vi "2P_AdapUprite_Linlin.vi"() -> ()   [LabVIEW 2015] (continued)
                                n2049 = call "waveformparamsv2.vi"("command"="add DO", "add DO"=w5235) -> ()  [unwired: 3 in, 3 out]
                                }
                                frame #2 {
                                n2050 = call "waveformsDObuffer.vi"("command"="get") -> ("DO wf out"=w5240:digitalwaveform[])  [unwired: 1 in]
                                n2051 = Build Array (concatenate)(w5240, w5237) -> (w5239:digitalwaveform[])
                                n2052 = call "waveformsDObuffer.vi"("DO wf in"=w5239, "command"="set") -> ()  [unwired: 1 out]
                                }
                                }
                                }
                                frame 0 {
                                n2053 = stacked-sequence {
                                seq-local: [w5248 _ _] -> [_ w5256 w5273]
                                tunnel: w5245 -> [_ _ _]
                                tunnel: w5244 -> [_ _ _]
                                tunnel: w5243 -> [_ w5253 _]
                                tunnel: w5242 -> [_ _ w5272]
                                frame #0 {
                                n2054 = call "configuration_2P_Linlin.vi"("command"="get") -> ("config out"=w5246:T14)  [unwired: 2 in, 1 out]
                                n2055 = Unbundle By Name(w5246) -> ("LT timestamp"=w5249:u32)
                                n2056 = call "2pparameters.vi"("command"="get") -> ("params out"=w5252:T12)  [unwired: 1 in]
                                n2057 = Unbundle By Name(w5252) -> ("aDO"=w5250:u32[])
                                n2058 = Search 1D Array(1D array=w5250, element=w5249) -> (index of element=w5248:i32)  [unwired: 1 in]
                                }
                                frame #1 {
                                n2059 = local read "Measurement"() -> (w5255:T4)
                                n2060 = To Unsigned Long Integer(number=w5255) -> (unsigned 32bit integer=w5254:u32)
                                n2061 = case shown="5..7" w5254 {
                                tunnel: w5256 -> [_ w5260]
                                tunnel: w5253 -> [_ w5257]
                                frame 0..4, Default {
                                }
                                frame 5..7 {
                                n2062 = Index Array(array=w5257, index=0) -> (element=w5258:T21)
                                n2063 = call "waveformparamsv2.vi"("command"="get") -> ("Params out"=w5263:T17)  [unwired: 4 in, 2 out]
                                n2064 = in-place {
                                in-place-border: w5260 -> [w5267]
                                in-place-border: w5258 -> [w5265]
                                n2065 = in-place-cluster #43(w5263) -> ("DO parameters"=w5268:T20)
                                n2066 = in-place {
                                in-place-border: w5265 -> [w5269]
                                n2067 = in-place-array #44(w5268, w5267) -> ()  [unwired: 1 out]
                                n2068 = in-place-array #44(w5269) -> (w5266:T20)  [unwired: 1 out]
                                }
                                n2069 = in-place-cluster #43("DO parameters"=w5266) -> (w5261:T17)
                                }
                                n2070 = call "waveformparamsv2.vi"("command"="set", "Params in"=w5261) -> ()  [unwired: 3 in, 3 out]
                                }
                                }
                                }
                                frame #2 {
                                n2071 = local read "Measurement"() -> (w5271:T4)
                                n2072 = To Unsigned Long Integer(number=w5271) -> (unsigned 32bit integer=w5270:u32)
                                n2073 = case shown="5..7" w5270 {
                                tunnel: w5273 -> [_ w5277]
                                tunnel: w5272 -> [_ w5275]
                                frame 0..4, Default {
                                }
                                frame 5..7 {
                                n2074 = Index Array(array=w5275, index=0) -> (element=w5274:digitalwaveform)
                                n2075 = call "waveformsDObuffer.vi"("command"="get") -> ("DO wf out"=w5279:digitalwaveform[])  [unwired: 1 in]
                                n2076 = Replace Array Subset(array=w5279, new element=w5274, index=w5277) -> (w5281:digitalwaveform[])
                                n2077 = call "waveformsDObuffer.vi"("DO wf in"=w5281, "command"="set") -> ()  [unwired: 1 out]
                                }
                                }
                                }
                                }
                                }
                                }
                              }
                              frame #4 {
                                n2078 = call "Used AO lines.vi"() -> ("used AO names"=w5284:string[], "used AO lines"=w5282:tag[])  [unwired: 2 in]
                                n2079 = control-ref of="Analog Lines Plot"() -> (w5283:refnum<vi>)
                                n2080 = control-ref of="Digital Lines Plot"() -> (w5285:refnum<vi>)
                                n2081 = call "Used DO lines.vi"() -> ("used DO names"=w5286:string[], "used DO lines"=w5287:tag[])  [unwired: 2 in]
                                n2082 = local write "Analog Used Lines"(w5282) -> ()
                                n2083 = local write "Analog Used Names"(w5284) -> ()
                                n2084 = local write "Digital Used Lines"(w5287) -> ()
                                n2085 = local write "Digital Used Names"(w5286) -> ()
                                n2086 = call "prepDOWaveplot.vi"("DigitalGraph in"=w5285, "used DO names"=w5286) -> ()  [unwired: 1 in]
                                n2087 = call "prepAOWaveplot.vi"("WaveformGraph in"=w5283, "Analog Used Names"=w5284) -> ()  [unwired: 1 in]
                              }
                              frame #5 {
                                # "source of crashing?"
                                n2088 = local read "Meastab"() -> (w5302:enum32{"X-Y Image", "Linescan", "Timetrace"})
                                n2089 = property on="refwf" class="Ring (strict)"() -> ("RingText.Text"=w5299:string)  [unwired: 2 in, 2 out]
                                n2090 = case shown="\"Timetrace\"" w5302 {
                                tunnel: [w5304 w5305] -> w5303
                                frame "X-Y Image", Default {
                                n2091 = local read "Sampling rate"() -> (w5304:dbl)
                                }
                                frame "Timetrace" {
                                n2092 = local read "srateAODOtt"() -> (w5305:dbl)
                                }
                                }
                                n2093 = call "waveformsAObuffer.vi"("command"="get") -> ("AO wf out"=w5290:waveform(dbl)[])  [unwired: 1 in]
                                n2094 = local read "wavdet"() -> (w5300:bool)
                                n2095 = call "waveformsDObuffer.vi"("command"="get") -> ("DO wf out"=w5294:digitalwaveform[])  [unwired: 1 in]
                                n2096 = call "correctwaveformsizetemp.vi"("new sampling frequency (Hz)"=w5303, "start"=FALSE, "reference waveforms to"=w5299, "Analog waveforms in"=w5290, "stop"=TRUE, "Digital waveforms in"=w5294) -> ("analog wf out"=w5296:waveform(dbl)[], "Digital wf out"=w5298:digitalwaveform[], "measpoints"=w5301:i32)
                                n2097 = local write "Analog Lines Plot"(w5296) -> ()
                                n2098 = call "GetNumCamFramesv2.vi"("Digital Waveform Graph"=w5298) -> ("Numeric"=w5297:i32)  [unwired: 10 in]
                                n2099 = local write "Digital Lines Plot"(w5298) -> ()
                                n2100 = call "waveformsDObuffer.vi"("DO wf in"=w5298, "command"="set") -> ()  [unwired: 1 out]
                                n2101 = call "waveformsAObuffer.vi"("AO wf in"=w5296, "command"="set") -> ()  [unwired: 1 out]
                                n2102 = local write "Total Camera Frames"(w5297) -> ()
                                n2103 = case shown="True" w5300 {
                                tunnel: w5301 -> [_ w5306]
                                frame False {
                                }
                                frame True {
                                n2104 = local write "# of frames"(w5306) -> ()
                                }
                                }
                              }
                            }
                          }
                          frame #9 {
                            w5316 = FALSE ("Value (Signaling)")
                            # "Save parameters, reset system..."
                            n2105 = local read "save\ndata"() -> (w5311:bool)
                            n2106 = case shown="True" w5311 {
                              tunnel: w5310 -> [_ w5323]
                              frame False {
                              }
                              frame True {
                                n2107 = call "closebinaryfiles.vi"() -> ()  [unwired: 12 in]
                                n2108 = local read "filename prefix"() -> (w5324:string)
                                n2109 = local read "data dir"() -> (w5325:path)
                                n2110 = disable-structure shown="Disabled" {
                                disable-tunnel: w5324 -> [w5328 _]
                                disable-tunnel: w5325 -> [w5327 _]
                                disable-tunnel: w5323 -> [w5326 _]
                                frame Disabled {
                                n2111 = call "saveparams.vi"("timestamp"=w5326, "filename prefix in"=w5328, "data dir in"=w5327) -> ()  [unwired: 1 in]
                                }
                                frame Enabled {
                                }
                                }
                                n2112 = call "saveparams_andscanpattern.vi"("timestamp"=w5323, "filename prefix in"=w5324, "data dir in"=w5325) -> ()  [unwired: 1 in]
                              }
                            }
                            n2113 = call "2pparameters.vi"("command"="get") -> ("params out"=w5307:T12)  [unwired: 1 in]
                            n2114 = Unbundle By Name(w5307) -> ("auto OD"=w5308:bool)
                            n2115 = case shown="True" w5308 {
                              frame False {
                              }
                              frame True {
                                n2116 = call "configuration_2P_Linlin.vi"("command"="get") -> ("config out"=w5317:T14)  [unwired: 2 in, 1 out]
                                n2117 = call "2pparameters.vi"("command"="get") -> ("params out"=w5322:T12)  [unwired: 1 in]
                                n2118 = Unbundle By Name(w5317) -> ("contour OD"=w5319:u16)
                                n2119 = Unbundle By Name(w5322) -> ("ODfilt"=w5320:u16)
                                n2120 = call "filterwheelcontrol_nothorlabslib.vi"("Current OD filt"=w5319, "New ODfilt"=w5320) -> ()  [unwired: 1 in]
                              }
                            }
                            n2121 = property on="Start" class="Bool (strict)"("Val(Sgnl)"=w5316) -> ()  [unwired: 2 in, 2 out]
                            n2122 = property on="Start" class="Bool (strict)"("Visible"=TRUE, "DisabledEnum"=T7."Enabled" ("Disabled")) -> ()  [unwired: 2 in, 2 out]
                            n2123 = property on="Stop" class="Bool (strict)"("Val(Sgnl)"=w5316) -> ()  [unwired: 2 in, 2 out]
                            n2124 = property on="Stop" class="Bool (strict)"("Visible"=FALSE, "DisabledEnum"=T7."Disabled" ("Disabled")) -> ()  [unwired: 2 in, 2 out]
                          }
                          frame #10 {
                            w5331 = T24 2 items=["no dialog", "OK message", "continue or stop message", "OK message + warnings", "continue/stop + warnings"] ("type of dialog (OK msg:1)")
                            # "Error Handling"
                            n2125 = call "displayerrors.vi"() -> ("error IO"=w5332:errorcluster)
                            n2126 = call <vilib>:"General Error Handler.vi"("type of dialog (OK msg:1)"=w5331, "error in (no error)"=w5332) -> ("error out"=w5330:errorcluster)  [unwired: 9 in, 4 out]
                            n2127 = call <vilib>:"Clear Errors.vi"("error in (no error)"=w5330) -> ("error out"=w5329:errorcluster)  [unwired: 5 in, 1 out]
                            n2128 = call "seterrors.vi"("error IO"=w5329) -> ()
                          }
                        }
                      }
                    }
                  }
                  frame "Lifetime (point)" {
                    # "Not really used"
                    # "Disabled for conversion to 64 bit"
                    n2129 = disable-structure shown="Disabled" {
                      frame Disabled {
                        n2130 = stacked-sequence {
                          frame #0 {
                            w5353 = 0.1 ("Y Scale.Range:Minimum")
                            w5354 = 0.0 ("X Scale.Range:Minimum")
                            # "get from syncrate"
                            n2131 = local read item#-1() -> (w5338)
                            n2132 = local read "Vx-ref"() -> (w5350:dbl)
                            n2133 = local read "Vy-ref"() -> (w5351:dbl)
                            n2134 = call "2pparameters.vi"("command"="get") -> ("params out"=w5336:T12)  [unwired: 1 in]
                            n2135 = Scale By Power Of 2(n=w5338, x=1.0 ("Y Scale.Range:Minimum")) -> (x*2^n=w5347:dbl)
                            n2136 = call "setposition.vi"("Vy"=w5351, "Vx"=w5350) -> ()  [unwired: 1 in]
                            n2137 = Unbundle By Name(w5336) -> ("autoshutter"=w5337:bool, "aAS"=w5334:u32[])
                            n2138 = Multiply(x=3000.0 ("Y Scale.Range:Minimum"), y=w5347) -> (x*y=w5345:dbl)
                            n2139 = Compound Arithmetic op=MULTIPLY(12.5 ("x"), invert 3200.0 ("X Scale.Offset and Multiplier:Multiplier"), w5347) -> (w5346:dbl)
                            n2140 = case shown="True" w5337 {
                              tunnel: w5334 -> [_ w5363]
                              frame False {
                              }
                              frame True {
                                n2141 = call "shuttercontrol_multi.vi"("Autoshutter Chans"=w5363, "command"="open") -> ()  [unwired: 1 in, 1 out]
                              }
                            }
                            n2142 = call "lifetimeparameters.vi"("command"="get") -> ("Params out"=w5342:T22)  [unwired: 1 in]
                            n2143 = Bundle By Name(cluster=w5342, "Bin size"=w5338) -> (w5343:T22)
                            n2144 = call "lifetimeparameters.vi"("Params in"=w5343, "command"="set") -> ()  [unwired: 1 out]
                            n2145 = call "2pparameters.vi"("command"="get") -> ("params out"=w5358:T12)  [unwired: 1 in]
                            n2146 = Bundle By Name(cluster=w5358, "type"="Lifetime (point)") -> (w5356:T12)
                            n2147 = property on="Stop" class="Bool (strict)"("Visible"=TRUE, "DisabledEnum"=T7."Enabled" ("Disabled")) -> ()  [unwired: 2 in, 2 out]
                            n2148 = property on="Start" class="Bool (strict)"("Visible"=FALSE, "DisabledEnum"=T7."Disabled and Grayed Out" ("Disabled")) -> ()  [unwired: 2 in, 2 out]
                            n2149 = call "2pparameters.vi"("Params in"=w5356, "command"="set") -> ()  [unwired: 1 out]
                          }
                          frame #1 {
                            n2150 = call "setup.vi"() -> ()  [unwired: 1 in]
                          }
                          frame #2 {
                            # "main loop"
                            n2151 = call "lifetimeparameters.vi"("command"="get") -> ("Params out"=w5369:T22)  [unwired: 1 in]
                            n2152 = Unbundle By Name(w5369) -> ("devidx"=w5367:i32)
                            n2153 = for {
                              N: 10000 -> [_]
                              tunnel: [w5370] -> w5365 mode=indexing
                              i -> [w5370]
                            }
                            n2154 = while {
                              tunnel: w5367 -> [w5374]
                              tunnel: w5365 -> [w5371]
                              i -> [w5372]
                              stop <- w5376 stop-if-true
                              n2155 = Increment(x=w5372) -> (x+1=w5373:i32)
                              n2156 = dll-call lib="phlib.dll" fn="_PH_GetCountRate@8" label="PH_GetCountRate"("devidx"=w5374, "channel"=0) -> (w5375:i32)  [unwired: 5 in, 2 out]
                              n2157 = stacked-sequence {
                                seq-local: [_ _ w5382 _ _] -> [_ _ _ w5395 _]
                                seq-local: [_ _ w5381 _ _] -> [_ _ _ w5394 _]
                                seq-local: [_ w5380 _ _ _] -> [_ _ w5383 _ _]
                                tunnel: w5375 -> [_ _ _ w5402 _]
                                tunnel: w5371 -> [_ _ _ w5392 _]
                                frame #0 {
                                n2158 = call "start_binned.vi"() -> ()  [unwired: 1 in]
                                }
                                frame #1 {
                                n2159 = call "get-histogram.vi"() -> ("Histogram"=w5380:u32[])  [unwired: 1 out]
                                }
                                frame #2 {
                                n2160 = Search 1D Array(1D array=w5383, element=u32 0) -> (index of element=w5381:i32)  [unwired: 1 in]
                                n2161 = Multiply(x=w5381, y=0.99) -> (x*y=w5387:dbl)
                                n2162 = Array Subset(array=w5383, index=0, length=w5387) -> (w5390:u32[])
                                n2163 = Array Max & Min(array=w5390) -> (max index (indices)=w5384:i32)  [unwired: 3 out]
                                n2164 = Split 1D Array(array=w5390, index=w5384) -> (second subarray=w5386:u32[])  [unwired: 1 out]
                                n2165 = Array Max & Min(array=w5386) -> (min index (indices)=w5385:i32)  [unwired: 3 out]
                                n2166 = Split 1D Array(array=w5386, index=w5385) -> (first subarray=w5382:u32[])  [unwired: 1 out]
                                }
                                frame #3 {
                                n2167 = Array Size(array=w5395) -> (size(s)=w5397:i32)
                                n2168 = Array Subset(array=w5392, index=0, length=w5397) -> (w5396:i32[])
                                n2169 = Compound Arithmetic op=MULTIPLY(1000000000.0 ("value"), invert w5402, invert w5394, w5396) -> (w5393:dbl[])
                                n2170 = call <vilib>:"Exponential Fit.vi"("Y"=w5395, "X"=w5393) -> ("damping"=w5399:dbl)  [unwired: 8 in, 5 out]
                                n2171 = Divide(x=-1.0 ("y"), y=w5399) -> (x/y=w5403:dbl)
                                }
                                frame #4 {
                                n2172 = local read "downright"() -> (w5409:bool)
                                n2173 = local read "downleft"() -> (w5411:bool)
                                n2174 = local read "upright"() -> (w5407:bool)
                                n2175 = local read "upleft"() -> (w5405:bool)
                                n2176 = local read "down"() -> (w5410:bool)
                                n2177 = local read "right"() -> (w5408:bool)
                                n2178 = local read "left"() -> (w5412:bool)
                                n2179 = local read "up"() -> (w5406:bool)
                                n2180 = Compound Arithmetic op=OR(w5405, w5406, w5407, w5408, w5409, w5410, w5411, w5412) -> (w5404:bool)
                                n2181 = case shown="True" w5404 {
                                frame False {
                                }
                                frame True {
                                n2182 = stacked-sequence {
                                frame #0 {
                                n2183 = local read "downright"() -> (w5414:bool)
                                n2184 = local read "downleft"() -> (w5416:bool)
                                n2185 = local read "BigSmall"() -> (w5413:bool)
                                n2186 = local read "upright"() -> (w5418:bool)
                                n2187 = local read "upleft"() -> (w5421:bool)
                                n2188 = local read "down"() -> (w5417:bool)
                                n2189 = local read "right"() -> (w5419:bool)
                                n2190 = local read "left"() -> (w5415:bool)
                                n2191 = local read "up"() -> (w5420:bool)
                                n2192 = call "movestageparams.vi"("command"="get") -> ("Params out"=w5424:T23)  [unwired: 1 in]
                                n2193 = Bundle By Name(cluster=w5424, "upleft"=w5421, "up"=w5420, "upright"=w5418, "right"=w5419, "downright"=w5414, "down"=w5417, "downleft"=w5416, "left"=w5415, "Bigsmall"=w5413) -> (w5425:T23)
                                n2194 = call "movestageparams.vi"("Params in"=w5425, "command"="set") -> ()  [unwired: 1 out]
                                }
                                frame #1 {
                                n2195 = call "movestage.vi"() -> ()  [unwired: 12 in]
                                }
                                frame #2 {
                                w5426 = FALSE ("OK Button")
                                w5427 = FALSE ("OK Button")
                                n2196 = property on="down" class="Bool (strict)"("Value"=w5427) -> ()  [unwired: 2 in, 2 out]
                                n2197 = property on="up" class="Bool (strict)"("Value"=w5427) -> ()  [unwired: 2 in, 2 out]
                                n2198 = property on="right" class="Bool (strict)"("Value"=w5427) -> ()  [unwired: 2 in, 2 out]
                                n2199 = property on="left" class="Bool (strict)"("Value"=w5427) -> ()  [unwired: 2 in, 2 out]
                                n2200 = property on="upleft" class="Bool (strict)"("Value"=w5426) -> ()  [unwired: 2 in, 2 out]
                                n2201 = property on="upright" class="Bool (strict)"("Value"=w5426) -> ()  [unwired: 2 in, 2 out]
                                n2202 = property on="downleft" class="Bool (strict)"("Value"=w5426) -> ()  [unwired: 2 in, 2 out]
                                n2203 = property on="downright" class="Bool (strict)"("Value"=w5426) -> ()  [unwired: 2 in, 2 out]
                                }
                                }
                                }
                                }
                                }
                              }
                              n2204 = dll-call lib="phlib.dll" fn="_PH_GetCountRate@8" label="PH_GetCountRate"("devidx"=w5374, "channel"=1) -> (w5379:i32)  [unwired: 5 in, 2 out]
                              n2205 = local read "Stop"() -> (w5376:bool)
                              n2206 = local write "points recorded"(w5373) -> ()
                            }
                          }
                          frame #3 {
                            w5436 = FALSE ("Value (Signaling)")
                            n2207 = call "2pparameters.vi"("command"="get") -> ("params out"=w5430:T12)  [unwired: 1 in]
                            n2208 = Unbundle By Name(w5430) -> ("autoshutter"=w5431:bool, "aAS"=w5428:u32[])
                            n2209 = case shown="True" w5431 {
                              tunnel: w5428 -> [_ w5437]
                              frame False {
                              }
                              frame True {
                                n2210 = call "shuttercontrol_multi.vi"("Autoshutter Chans"=w5437, "command"="close") -> ()  [unwired: 1 in, 1 out]
                              }
                            }
                            n2211 = property on="Start" class="Bool (strict)"("Val(Sgnl)"=w5436) -> ()  [unwired: 2 in, 2 out]
                            n2212 = property on="Start" class="Bool (strict)"("Visible"=TRUE, "DisabledEnum"=T7."Enabled" ("Disabled")) -> ()  [unwired: 2 in, 2 out]
                            n2213 = property on="Stop" class="Bool (strict)"("Val(Sgnl)"=w5436) -> ()  [unwired: 2 in, 2 out]
                            n2214 = property on="Stop" class="Bool (strict)"("Visible"=FALSE, "DisabledEnum"=T7."Disabled" ("Disabled")) -> ()  [unwired: 2 in, 2 out]
                          }
                        }
                      }
                      frame Enabled {
                      }
                    }
                    n2215 = local write "64bit disabled"(TRUE ("64bit disabled")) -> ()
                  }
                }
              }
            }
          }
          event "avpp", "Angle ref", "xpixels ref", "Vx-min ref", "Vx-max ref", "ypixels ref", "Vy-min ref", "Vy-max ref", "ROI Type", "Sampling rate": Value Change {
            n2216 = event-data() -> ()  [unwired: 1 in, 6 out]
            n2217 = local read "avpp"() -> (w5456:i32)
            n2218 = local read "Angle ref"() -> (w5455:dbl)
            n2219 = local read "ROI Type"() -> (w5454:u16)
            n2220 = local read "xpixels ref"() -> (w5451:i32)
            n2221 = local read "Vx-min ref"() -> (w5450:dbl)
            n2222 = local read "Vx-max ref"() -> (w5449:dbl)
            n2223 = local read "ypixels ref"() -> (w5447:i32)
            n2224 = local read "Vy-min ref"() -> (w5448:dbl)
            n2225 = local read "Vy-max ref"() -> (w5444:dbl)
            n2226 = local read "Sampling rate"() -> (w5439:dbl)
            n2227 = local read "# of frames"() -> (w5443:i32)
            n2228 = local read "maxbufferAI"() -> (w5442:i32)
            n2229 = local read "Override AI buffer"() -> (w5440:bool)
            n2230 = call "2pparameters.vi"("command"="get") -> ("params out"=w5453:T12)  [unwired: 1 in]
            n2231 = Bundle By Name(cluster=w5453, "avpp"=w5456, "Angle Img"=w5455, "Xpixels Img"=w5451, "Vx-min Img"=w5450, "VX-max Img"=w5449, "Ypixels Img"=w5447, "Vy-min Img"=w5448, "Vy-max Img"=w5444, "srate"=w5439, "srate Img"=w5439, "measpoints"=w5443, "maxbufferAI"=w5442, "Drawing Mode"=w5454, "Vz-reset"=0.0, "AIoverride"=w5440) -> (w5445:T12)
            n2232 = call "2pparameters.vi"("Params in"=w5445, "command"="set") -> ()  [unwired: 1 out]
          }
          event "# of frames": Value Change {
            n2233 = event-data() -> ()  [unwired: 1 in, 6 out]
            n2234 = local read "Meastab"() -> (w5457:enum32{"X-Y Image", "Linescan", "Timetrace"})
            n2235 = case shown="\"Linescan\"" w5457 {
              frame "X-Y Image", Default {
                n2236 = local read "# of frames"() -> (w5458:i32)
                n2237 = call "2pparameters.vi"("command"="get") -> ("params out"=w5462:T12)  [unwired: 1 in]
                n2238 = Bundle By Name(cluster=w5462, "measpoints"=w5458) -> (w5459:T12)
                n2239 = call "2pparameters.vi"("Params in"=w5459, "command"="set") -> ()  [unwired: 1 out]
              }
              frame "Linescan" {
                n2240 = local read "srateAODOtt"() -> (w5472:dbl)
                n2241 = local read "# of frames"() -> (w5468:i32)
                n2242 = local read "refreshtime"() -> (w5474:dbl)
                n2243 = local read "bin"() -> (w5469:dbl)
                n2244 = call "tt_timeandsamples.vi"("bin"=w5469, "refreshtime"=w5474, "srateAODOtt"=w5472, "tot#ofsamples"=w5468) -> ("refreshrate"=w5471:dbl, "refreshbuffer"=w5470:i32, "timetracecycles"=w5467:i32)  [unwired: 5 in]
                n2245 = call "2pparameters.vi"("command"="get") -> ("params out"=w5464:T12)  [unwired: 1 in]
                n2246 = Bundle By Name(cluster=w5464, "measpoints"=w5468, "tt_cycles"=w5467, "refreshbuffer"=w5470, "refreshrate"=w5471) -> (w5466:T12)
                n2247 = Reciprocal(x=w5471) -> (1/x=w5473:dbl)
                n2248 = local write "refreshtime"(w5473) -> ()
                n2249 = call "2pparameters.vi"("Params in"=w5466, "command"="set") -> ()  [unwired: 1 out]
              }
              frame "Timetrace" {
                n2250 = local read "srateAODOtt"() -> (w5484:dbl)
                n2251 = local read "# of frames"() -> (w5480:i32)
                n2252 = local read "refreshtime"() -> (w5486:dbl)
                n2253 = local read "bin"() -> (w5481:dbl)
                n2254 = call "tt_timeandsamples.vi"("bin"=w5481, "refreshtime"=w5486, "srateAODOtt"=w5484, "tot#ofsamples"=w5480) -> ("refreshrate"=w5483:dbl, "refreshbuffer"=w5482:i32, "timetracecycles"=w5479:i32)  [unwired: 5 in]
                n2255 = call "2pparameters.vi"("command"="get") -> ("params out"=w5476:T12)  [unwired: 1 in]
                n2256 = Bundle By Name(cluster=w5476, "measpoints"=w5480, "tt_cycles"=w5479, "refreshbuffer"=w5482, "refreshrate"=w5483) -> (w5478:T12)
                n2257 = Reciprocal(x=w5483) -> (1/x=w5485:dbl)
                n2258 = local write "refreshtime"(w5485) -> ()
                n2259 = call "2pparameters.vi"("Params in"=w5478, "command"="set") -> ()  [unwired: 1 out]
              }
            }
          }
          event "srateAODOtt", "refreshtime", "Vx-ref", "Vy-ref", "Vx-min draw", "Vx-max draw", "Vy-min draw", "Vy-max draw", "bin": Value Change {
            n2260 = event-data() -> ()  [unwired: 1 in, 6 out]
            n2261 = local read "ypixels ref"() -> (w5518:i32)
            n2262 = local read "Vy-min draw"() -> (w5494:dbl)
            n2263 = local read "Vy-max draw"() -> (w5493:dbl)
            n2264 = local read "Vx-min draw"() -> (w5496:dbl)
            n2265 = local read "Vx-max draw"() -> (w5495:dbl)
            n2266 = local read "xpixels ref"() -> (w5492:i32)
            n2267 = local read "ROI Type"() -> (w5491:u16)
            n2268 = local read "Pel"() -> (w5490:dbl)
            n2269 = local read "srateAODOtt"() -> (w5500:dbl)
            n2270 = local read "# of frames"() -> (w5505:i32)
            n2271 = local read "refreshtime"() -> (w5498:dbl)
            n2272 = local read "bin"() -> (w5503:dbl)
            n2273 = local read "Override AI buffer"() -> (w5488:bool)
            n2274 = local read "finite samples"() -> (w5512:bool)
            n2275 = local read "srateAODOtt"() -> (w5487:dbl)
            n2276 = local read "srateAODOtt"() -> (w5506:dbl)
            n2277 = local read "continuous"() -> (w5511:bool)
            n2278 = local read "Angle ref"() -> (w5497:dbl)
            n2279 = local read "wavdet"() -> (w5513:bool)
            n2280 = local read "Vx-ref"() -> (w5508:dbl)
            n2281 = local read "Vy-ref"() -> (w5510:dbl)
            n2282 = local read "avpp"() -> (w5509:i32)
            n2283 = call "tt_timeandsamples.vi"("bin"=w5503, "refreshtime"=w5498, "srateAODOtt"=w5500, "tot#ofsamples"=w5505) -> ("refreshrate"=w5501:dbl, "refreshbuffer"=w5502:i32, "timetracecycles"=w5507:i32)  [unwired: 5 in]
            n2284 = local read "bin"() -> (w5504:dbl)
            n2285 = call "2pparameters.vi"("command"="get") -> ("params out"=w5516:T12)  [unwired: 1 in]
            n2286 = Bundle By Name(cluster=w5516, "Drawing Mode"=w5491, "measpoints"=w5505, "tt_cycles"=w5507, "refreshbuffer"=w5502, "refreshrate"=w5501, "Vx-ref"=w5508, "Vy-ref"=w5510, "srate"=w5487, "finite"=w5512, "cont"=w5511, "wavdet"=w5513, "avpp"=w5509, "srateAODO"=w5506, "bufferAI"=w5502, "bin"=w5504, "Angle Img"=w5497, "Vxminref"=w5496, "Vxmaxref"=w5495, "Vyminref"=w5494, "Vymaxref"=w5493, "Xpixels Img"=w5492, "Ypixels Img"=w5518, "Pel"=w5490, "Vz-reset"=0.0, "AIoverride"=w5488) -> (w5514:T12)
            n2287 = Reciprocal(x=w5501) -> (1/x=w5499:dbl)
            n2288 = local write "refreshtime"(w5499) -> ()
            n2289 = call "2pparameters.vi"("Params in"=w5514, "command"="set") -> ()  [unwired: 1 out]
          }
          event "Init": Value Change {
            # "Disabled for conversion to 64 bit"
            n2290 = event-data() -> ()  [unwired: 1 in, 6 out]
            n2291 = disable-structure shown="Disabled" {
              frame Disabled {
                n2292 = flat-sequence {
                  frame #0 {
                    n2293 = local read "Measurement"() -> (w5520:T4)
                    n2294 = case shown="\"Lifetime (scan)\", \"Lifetime (contour)\"" w5520 {
                      frame "X-Y-t movie", Default {
                      }
                      frame "Lifetime (point)" {
                        n2295 = stacked-sequence {
                          frame #0 {
                            n2296 = call "initialize.vi"("mode"=0) -> ()
                          }
                          frame #1 {
                            n2297 = call "calib.vi"() -> ()  [unwired: 1 in]
                          }
                        }
                      }
                      frame "Lifetime (scan)", "Lifetime (contour)" {
                        n2298 = stacked-sequence {
                          frame #0 {
                            n2299 = call "initialize.vi"("mode"=3) -> ()
                          }
                          frame #1 {
                            n2300 = call "calib.vi"() -> ()  [unwired: 1 in]
                          }
                        }
                      }
                    }
                  }
                  frame #1 {
                    n2301 = property on="Start" class="Bool (strict)"("Visible"=TRUE, "DisabledEnum"=T7."Enabled" ("Disabled")) -> ()  [unwired: 2 in, 2 out]
                    n2302 = property on="Init" class="Bool (strict)"("Visible"=FALSE, "DisabledEnum"=T7."Disabled and Grayed Out" ("Disabled"), "Value"=FALSE ("Init")) -> ()  [unwired: 2 in, 2 out]
                  }
                }
              }
              frame Enabled {
              }
            }
            n2303 = local write "64bit disabled"(TRUE ("64bit disabled")) -> ()
          }
          event "Measurement": Value Change {
            n2304 = event-data() -> ()  [unwired: 1 in, 5 out]
            n2305 = case shown="\"X-Y-t movie\"" "Measurement" {
              frame "X-Y-t movie" {
                w5535 = T7."Disabled" ("Disabled")
                w5534 = FALSE ("Visible")
                n2306 = call "2pparameters.vi"("command"="get") -> ("params out"=w5545:T12)  [unwired: 1 in]
                n2307 = local write "graphtab"(T8."image" ("graphtab")) -> ()
                n2308 = local write "Save tab"(enum32{"withsave", "withoutsave"}."withsave" ("Save tab")) -> ()
                n2309 = Bundle By Name(cluster=w5545, "type"="X-Y-t movie") -> (w5543:T12)
                n2310 = call "2pparameters.vi"("Params in"=w5543, "command"="set") -> ()  [unwired: 1 out]
                n2311 = property on="refreshtime" class="DigNum (strict)"("Visible"=FALSE, "DisabledEnum"=T7."Disabled and Grayed Out" ("Disabled")) -> ()  [unwired: 2 in, 2 out]
                n2312 = property on="Start" class="Bool (strict)"("Visible"=TRUE, "DisabledEnum"=T7."Enabled" ("Disabled")) -> ()  [unwired: 2 in, 2 out]
                n2313 = property on="Init" class="Bool (strict)"("Visible"=FALSE, "DisabledEnum"=T7."Disabled and Grayed Out" ("Disabled"), "Value"=FALSE ("Init")) -> ()  [unwired: 2 in, 2 out]
                n2314 = property on="ttt" class="Enum (strict)"("Visible"=FALSE) -> ()  [unwired: 2 in, 2 out]
                n2315 = property on="# of frames" class="DigNum (strict)"("DisabledEnum"=T7."Enabled" ("Disabled"), "Caption.Text"="# of frames") -> ()  [unwired: 2 in, 2 out]
                n2316 = property on="continuous" class="Bool (strict)"("Visible"=TRUE, "DisabledEnum"=T7."Enabled" ("Disabled")) -> ()  [unwired: 2 in, 2 out]
                n2317 = property on="finite samples" class="Bool (strict)"("Visible"=TRUE, "DisabledEnum"=T7."Enabled" ("Disabled")) -> ()  [unwired: 2 in, 2 out]
                n2318 = property on="avpp" class="DigNum (strict)"("Visible"=TRUE, "DisabledEnum"=T7."Enabled" ("Disabled")) -> ()  [unwired: 2 in, 2 out]
                n2319 = property on="srateAODOtt" class="DigNum (strict)"("Visible"=FALSE, "DisabledEnum"=T7."Disabled" ("Disabled")) -> ()  [unwired: 2 in, 2 out]
                n2320 = local write "save\ndata"(TRUE ("save\ndata")) -> ()
                n2321 = property on="finite samples" class="Bool (strict)"("Val(Sgnl)"=TRUE ("continuous for display")) -> ()  [unwired: 2 in, 2 out]
                n2322 = property on="continuous" class="Bool (strict)"("Value"=FALSE ("continuous for display")) -> ()  [unwired: 2 in, 2 out]
                n2323 = property on="Current Average" class="DigNum (strict)"("Visible"=TRUE, "DisabledEnum"=T7."Enabled" ("Disabled")) -> ()  [unwired: 2 in, 2 out]
                n2324 = property on="img_CH1" class="IntGraph (strict)"("ZScale.Maximum"=7.0 ("Z Scale.Range:Maximum")) -> ()  [unwired: 2 in, 2 out]
                n2325 = property on="Sampling rate" class="DigNum (strict)"("Visible"=TRUE, "DisabledEnum"=T7."Enabled" ("Disabled")) -> ()  [unwired: 2 in, 2 out]
                n2326 = property on="Pel" class="DigNum (strict)"("Visible"=w5534, "DisabledEnum"=w5535) -> ()  [unwired: 2 in, 2 out]
                n2327 = property on="bin" class="DigNum (strict)"("Visible"=w5534, "DisabledEnum"=w5535) -> ()  [unwired: 2 in, 2 out]
                "Meastab" <- enum32{"X-Y Image", "Linescan", "Timetrace"}."X-Y Image" ("Meastab")
                "Zscantab" <- enum32{"withzscan", "withoutzscan", "lifetime"}."withoutzscan" ("Zscantab")
              }
              frame "X-Y-Z stack" {
                w5572 = T7."Disabled" ("Disabled")
                w5571 = FALSE ("Visible")
                n2328 = call "2pparameters.vi"("command"="get") -> ("params out"=w5582:T12)  [unwired: 1 in]
                n2329 = call "2pparameters.vi"("command"="get") -> ("params out"=w5586:T12)  [unwired: 1 in]
                n2330 = Bundle By Name(cluster=w5582, "type"="X-Y-Z stack") -> (w5580:T12)
                n2331 = Unbundle By Name(w5586) -> ("motorref"=w5585:refnum<k7>)
                n2332 = call "2pparameters.vi"("Params in"=w5580, "command"="set") -> ()  [unwired: 1 out]
                n2333 = local write "Zscantab"(enum32{"withzscan", "withoutzscan", "lifetime"}."withzscan" ("Zscantab")) -> ()
                n2334 = local write "Meastab"(enum32{"X-Y Image", "Linescan", "Timetrace"}."X-Y Image" ("Meastab")) -> ()
                n2335 = invoke class="MG17Motor" method="GetPosition"(reference=w5585, "lChanID"=0, "pfPosition"=sgl 0.0) -> ("pfPosition"=w5597:sgl)  [unwired: 2 in, 4 out]
                n2336 = property on="refreshtime" class="DigNum (strict)"("Visible"=FALSE, "DisabledEnum"=T7."Disabled and Grayed Out" ("Disabled")) -> ()  [unwired: 2 in, 2 out]
                n2337 = property on="Start" class="Bool (strict)"("Visible"=TRUE, "DisabledEnum"=T7."Enabled" ("Disabled")) -> ()  [unwired: 2 in, 2 out]
                n2338 = property on="Init" class="Bool (strict)"("Visible"=FALSE, "DisabledEnum"=T7."Disabled and Grayed Out" ("Disabled"), "Value"=FALSE ("Init")) -> ()  [unwired: 2 in, 2 out]
                n2339 = property on="ttt" class="Enum (strict)"("Visible"=FALSE) -> ()  [unwired: 2 in, 2 out]
                n2340 = Multiply(x=w5597, y=1000.0) -> (x*y=w5596:dbl)
                n2341 = local write "Actual Z position"(w5596) -> ()
                n2342 = local write "Save tab"(enum32{"withsave", "withoutsave"}."withsave" ("Save tab")) -> ()
                n2343 = property on="finite samples" class="Bool (strict)"("Visible"=FALSE, "DisabledEnum"=T7."Disabled and Grayed Out" ("Disabled")) -> ()  [unwired: 2 in, 2 out]
                n2344 = property on="avpp" class="DigNum (strict)"("Visible"=TRUE, "DisabledEnum"=T7."Enabled" ("Disabled")) -> ()  [unwired: 2 in, 2 out]
                n2345 = property on="continuous" class="Bool (strict)"("Visible"=FALSE, "DisabledEnum"=T7."Disabled and Grayed Out" ("Disabled")) -> ()  [unwired: 2 in, 2 out]
                n2346 = property on="img_CH1" class="IntGraph (strict)"("ZScale.Maximum"=7.0 ("Z Scale.Range:Maximum")) -> ()  [unwired: 2 in, 2 out]
                n2347 = property on="srateAODOtt" class="DigNum (strict)"("Visible"=FALSE, "DisabledEnum"=T7."Disabled" ("Disabled")) -> ()  [unwired: 2 in, 2 out]
                n2348 = property on="Pel" class="DigNum (strict)"("Visible"=w5571, "DisabledEnum"=w5572) -> ()  [unwired: 2 in, 2 out]
                n2349 = property on="bin" class="DigNum (strict)"("Visible"=w5571, "DisabledEnum"=w5572) -> ()  [unwired: 2 in, 2 out]
                n2350 = property on="Current Average" class="DigNum (strict)"("Visible"=TRUE, "DisabledEnum"=T7."Enabled" ("Disabled")) -> ()  [unwired: 2 in, 2 out]
                n2351 = property on="# of frames" class="DigNum (strict)"("Caption.Text"="# of slices", "DisabledEnum"=T7."Disabled and Grayed Out" ("Disabled")) -> ()  [unwired: 2 in, 2 out]
                n2352 = local write "save\ndata"(TRUE ("save\ndata")) -> ()
                n2353 = property on="finite samples" class="Bool (strict)"("Val(Sgnl)"=TRUE ("continuous for display")) -> ()  [unwired: 2 in, 2 out]
                n2354 = property on="continuous" class="Bool (strict)"("Value"=FALSE ("continuous for display")) -> ()  [unwired: 2 in, 2 out]
                n2355 = property on="Sampling rate" class="DigNum (strict)"("Visible"=TRUE, "DisabledEnum"=T7."Enabled" ("Disabled")) -> ()  [unwired: 2 in, 2 out]
              }
              frame "X-Y-Z-t movie" {
                w5616 = T7."Disabled" ("Disabled")
                w5615 = FALSE ("Visible")
                n2356 = property on="# of frames" class="DigNum (strict)"("DisabledEnum"=T7."Enabled" ("Disabled")) -> ()  [unwired: 2 in, 2 out]
                n2357 = property on="Current Average" class="DigNum (strict)"("Visible"=TRUE, "DisabledEnum"=T7."Enabled" ("Disabled")) -> ()  [unwired: 2 in, 2 out]
                n2358 = property on="avpp" class="DigNum (strict)"("Visible"=TRUE, "DisabledEnum"=T7."Enabled" ("Disabled")) -> ()  [unwired: 2 in, 2 out]
                n2359 = local write "Save tab"(enum32{"withsave", "withoutsave"}."withsave" ("Save tab")) -> ()
                n2360 = local write "Zscantab"(enum32{"withzscan", "withoutzscan", "lifetime"}."withzscan" ("Zscantab")) -> ()
                n2361 = local write "Meastab"(enum32{"X-Y Image", "Linescan", "Timetrace"}."X-Y Image" ("Meastab")) -> ()
                n2362 = property on="Start" class="Bool (strict)"("Visible"=TRUE, "DisabledEnum"=T7."Enabled" ("Disabled")) -> ()  [unwired: 2 in, 2 out]
                n2363 = property on="refreshtime" class="DigNum (strict)"("Visible"=FALSE, "DisabledEnum"=T7."Disabled and Grayed Out" ("Disabled")) -> ()  [unwired: 2 in, 2 out]
                n2364 = property on="Init" class="Bool (strict)"("Visible"=FALSE, "DisabledEnum"=T7."Disabled and Grayed Out" ("Disabled"), "Value"=FALSE ("Init")) -> ()  [unwired: 2 in, 2 out]
                n2365 = property on="ttt" class="Enum (strict)"("Visible"=FALSE) -> ()  [unwired: 2 in, 2 out]
                n2366 = call "2pparameters.vi"("command"="get") -> ("params out"=w5626:T12)  [unwired: 1 in]
                n2367 = Bundle By Name(cluster=w5626, "type"="X-Y-Z-t movie") -> (w5624:T12)
                n2368 = property on="continuous" class="Bool (strict)"("Visible"=TRUE, "DisabledEnum"=T7."Enabled" ("Disabled")) -> ()  [unwired: 2 in, 2 out]
                n2369 = property on="finite samples" class="Bool (strict)"("Visible"=TRUE, "DisabledEnum"=T7."Enabled" ("Disabled")) -> ()  [unwired: 2 in, 2 out]
                n2370 = call "2pparameters.vi"("Params in"=w5624, "command"="set") -> ()  [unwired: 1 out]
                n2371 = property on="srateAODOtt" class="DigNum (strict)"("Visible"=FALSE, "DisabledEnum"=T7."Disabled" ("Disabled")) -> ()  [unwired: 2 in, 2 out]
                n2372 = local write "save\ndata"(TRUE ("save\ndata")) -> ()
                n2373 = property on="img_CH1" class="IntGraph (strict)"("ZScale.Maximum"=7.0 ("Z Scale.Range:Maximum")) -> ()  [unwired: 2 in, 2 out]
                n2374 = property on="continuous" class="Bool (strict)"("Value"=FALSE ("continuous for display")) -> ()  [unwired: 2 in, 2 out]
                n2375 = property on="finite samples" class="Bool (strict)"("Value"=TRUE ("continuous for display")) -> ()  [unwired: 2 in, 2 out]
                n2376 = property on="Sampling rate" class="DigNum (strict)"("Visible"=TRUE, "DisabledEnum"=T7."Enabled" ("Disabled")) -> ()  [unwired: 2 in, 2 out]
                n2377 = property on="Pel" class="DigNum (strict)"("Visible"=w5615, "DisabledEnum"=w5616) -> ()  [unwired: 2 in, 2 out]
                n2378 = property on="bin" class="DigNum (strict)"("Visible"=w5615, "DisabledEnum"=w5616) -> ()  [unwired: 2 in, 2 out]
              }
              frame "linescan" {
                w5651 = T7."Enabled" ("Disabled")
                w5650 = TRUE ("Visible")
                w5653 = T7."Enabled" ("Disabled")
                w5652 = TRUE ("Visible")
                n2379 = local write "Meastab"(enum32{"X-Y Image", "Linescan", "Timetrace"}."Linescan" ("Meastab")) -> ()
                n2380 = property on="Current Average" class="DigNum (strict)"("Visible"=TRUE, "DisabledEnum"=T7."Enabled" ("Disabled")) -> ()  [unwired: 2 in, 2 out]
                n2381 = property on="ttt" class="Enum (strict)"("Visible"=FALSE) -> ()  [unwired: 2 in, 2 out]
                n2382 = local write "Save tab"(enum32{"withsave", "withoutsave"}."withsave" ("Save tab")) -> ()
                n2383 = local write "Zscantab"(enum32{"withzscan", "withoutzscan", "lifetime"}."withoutzscan" ("Zscantab")) -> ()
                n2384 = property on="refreshtime" class="DigNum (strict)"("Visible"=FALSE, "DisabledEnum"=T7."Disabled and Grayed Out" ("Disabled")) -> ()  [unwired: 2 in, 2 out]
                n2385 = property on="continuous" class="Bool (strict)"("Value"=FALSE ("continuous for display")) -> ()  [unwired: 2 in, 2 out]
                n2386 = property on="finite samples" class="Bool (strict)"("Value"=TRUE ("continuous for display")) -> ()  [unwired: 2 in, 2 out]
                n2387 = local write "save\ndata"(TRUE ("save\ndata")) -> ()
                n2388 = property on="Start" class="Bool (strict)"("Visible"=TRUE, "DisabledEnum"=T7."Enabled" ("Disabled")) -> ()  [unwired: 2 in, 2 out]
                n2389 = property on="Init" class="Bool (strict)"("Visible"=FALSE, "DisabledEnum"=T7."Disabled and Grayed Out" ("Disabled"), "Value"=FALSE ("Init")) -> ()  [unwired: 2 in, 2 out]
                n2390 = call "2pparameters.vi"("command"="get") -> ("params out"=w5662:T12)  [unwired: 1 in]
                n2391 = Bundle By Name(cluster=w5662, "type"="linescan") -> (w5660:T12)
                n2392 = property on="# of frames" class="DigNum (strict)"("DisabledEnum"=T7."Enabled" ("Disabled"), "Caption.Text"="# of lines") -> ()  [unwired: 2 in, 2 out]
                n2393 = property on="continuous" class="Bool (strict)"("Visible"=TRUE, "DisabledEnum"=T7."Enabled" ("Disabled")) -> ()  [unwired: 2 in, 2 out]
                n2394 = property on="avpp" class="DigNum (strict)"("Visible"=TRUE, "DisabledEnum"=T7."Enabled" ("Disabled")) -> ()  [unwired: 2 in, 2 out]
                n2395 = property on="finite samples" class="Bool (strict)"("Visible"=TRUE, "DisabledEnum"=T7."Enabled" ("Disabled")) -> ()  [unwired: 2 in, 2 out]
                n2396 = property on="srateAODOtt" class="DigNum (strict)"("Visible"=TRUE, "DisabledEnum"=T7."Enabled" ("Disabled")) -> ()  [unwired: 2 in, 2 out]
                n2397 = call "2pparameters.vi"("Params in"=w5660, "command"="set") -> ()  [unwired: 1 out]
                n2398 = property on="Pel" class="DigNum (strict)"("Visible"=w5652, "DisabledEnum"=w5653) -> ()  [unwired: 2 in, 2 out]
                n2399 = property on="bin" class="DigNum (strict)"("Visible"=w5652, "DisabledEnum"=w5653) -> ()  [unwired: 2 in, 2 out]
                n2400 = property on="Sampling rate" class="DigNum (strict)"("Visible"=FALSE, "DisabledEnum"=T7."Disabled" ("Disabled")) -> ()  [unwired: 2 in, 2 out]
                n2401 = property on="Pel" class="DigNum (strict)"("Visible"=w5650, "DisabledEnum"=w5651) -> ()  [unwired: 2 in, 2 out]
                n2402 = property on="bin" class="DigNum (strict)"("Visible"=w5650, "DisabledEnum"=w5651) -> ()  [unwired: 2 in, 2 out]
              }
              frame "Timetrace" {
                w5688 = T7."Enabled" ("Disabled")
                w5687 = TRUE ("Visible")
                n2403 = call "2pparameters.vi"("command"="get") -> ("params out"=w5693:T12)  [unwired: 1 in]
                n2404 = local write "Meastab"(enum32{"X-Y Image", "Linescan", "Timetrace"}."Timetrace" ("Meastab")) -> ()
                n2405 = Unbundle By Name(w5693) -> ("Angle draw"=w5695:dbl)
                n2406 = local write "Zscantab"(enum32{"withzscan", "withoutzscan", "lifetime"}."withoutzscan" ("Zscantab")) -> ()
                n2407 = property on="# of frames" class="DigNum (strict)"("DisabledEnum"=T7."Enabled" ("Disabled"), "Caption.Text"="# of samples") -> ()  [unwired: 2 in, 2 out]
                n2408 = property on="refreshtime" class="DigNum (strict)"("Visible"=TRUE, "DisabledEnum"=T7."Enabled" ("Disabled")) -> ()  [unwired: 2 in, 2 out]
                n2409 = property on="avpp" class="DigNum (strict)"("Visible"=FALSE, "DisabledEnum"=T7."Disabled and Grayed Out" ("Disabled")) -> ()  [unwired: 2 in, 2 out]
                n2410 = property on="Current Average" class="DigNum (strict)"("Visible"=FALSE, "DisabledEnum"=T7."Disabled and Grayed Out" ("Disabled")) -> ()  [unwired: 2 in, 2 out]
                n2411 = local write "Angle drawing"(w5695) -> ()
                n2412 = property on="ttt" class="Enum (strict)"("Visible"=TRUE) -> ()  [unwired: 2 in, 2 out]
                n2413 = property on="continuous" class="Bool (strict)"("Visible"=TRUE, "DisabledEnum"=T7."Enabled" ("Disabled")) -> ()  [unwired: 2 in, 2 out]
                n2414 = property on="finite samples" class="Bool (strict)"("Visible"=TRUE, "DisabledEnum"=T7."Enabled" ("Disabled")) -> ()  [unwired: 2 in, 2 out]
                n2415 = local write "save\ndata"(TRUE ("save\ndata")) -> ()
                n2416 = property on="finite samples" class="Bool (strict)"("Val(Sgnl)"=TRUE ("continuous for display")) -> ()  [unwired: 2 in, 2 out]
                n2417 = property on="continuous" class="Bool (strict)"("Value"=FALSE ("continuous for display")) -> ()  [unwired: 2 in, 2 out]
                n2418 = local write "Save tab"(enum32{"withsave", "withoutsave"}."withsave" ("Save tab")) -> ()
                n2419 = property on="srateAODOtt" class="DigNum (strict)"("Visible"=TRUE, "DisabledEnum"=T7."Enabled" ("Disabled")) -> ()  [unwired: 2 in, 2 out]
                n2420 = call "2pparameters.vi"("command"="get") -> ("params out"=w5700:T12)  [unwired: 1 in]
                n2421 = property on="Start" class="Bool (strict)"("Visible"=TRUE, "DisabledEnum"=T7."Enabled" ("Disabled")) -> ()  [unwired: 2 in, 2 out]
                n2422 = property on="Init" class="Bool (strict)"("Visible"=FALSE, "DisabledEnum"=T7."Disabled and Grayed Out" ("Disabled"), "Value"=FALSE ("Init")) -> ()  [unwired: 2 in, 2 out]
                n2423 = Bundle By Name(cluster=w5700, "type"="Timetrace") -> (w5698:T12)
                n2424 = property on="Sampling rate" class="DigNum (strict)"("Visible"=FALSE, "DisabledEnum"=T7."Disabled" ("Disabled")) -> ()  [unwired: 2 in, 2 out]
                n2425 = property on="Pel" class="DigNum (strict)"("Visible"=w5687, "DisabledEnum"=w5688) -> ()  [unwired: 2 in, 2 out]
                n2426 = property on="bin" class="DigNum (strict)"("Visible"=w5687, "DisabledEnum"=w5688) -> ()  [unwired: 2 in, 2 out]
                n2427 = call "2pparameters.vi"("Params in"=w5698, "command"="set") -> ()  [unwired: 1 out]
              }
              frame "Lifetime (point)" {
                w5721 = T7."Enabled" ("Disabled")
                w5720 = TRUE ("Visible")
                n2428 = property on="Pel" class="DigNum (strict)"("Visible"=w5720, "DisabledEnum"=w5721) -> ()  [unwired: 2 in, 2 out]
                n2429 = property on="bin" class="DigNum (strict)"("Visible"=w5720, "DisabledEnum"=w5721) -> ()  [unwired: 2 in, 2 out]
                n2430 = property on="ttt" class="Enum (strict)"("Visible"=FALSE) -> ()  [unwired: 2 in, 2 out]
                n2431 = local write "Zscantab"(enum32{"withzscan", "withoutzscan", "lifetime"}."lifetime" ("Zscantab")) -> ()
                n2432 = local write "graphtab"(T8."Lifetime" ("graphtab")) -> ()
                n2433 = local write "Meastab"(enum32{"X-Y Image", "Linescan", "Timetrace"}."Timetrace" ("Meastab")) -> ()
                n2434 = call "lifetimeparameters.vi"("command"="get") -> ("Params out"=w5728:T22)  [unwired: 1 in]
                n2435 = Unbundle By Name(w5728) -> ("initialized"=w5729:bool)
                n2436 = property on="srateAODOtt" class="DigNum (strict)"("Visible"=TRUE, "DisabledEnum"=T7."Enabled" ("Disabled")) -> ()  [unwired: 2 in, 2 out]
                n2437 = case shown="False" w5729 {
                  frame False {
                    n2438 = property on="Init" class="Bool (strict)"("Visible"=TRUE, "DisabledEnum"=T7."Enabled" ("Disabled")) -> ()  [unwired: 2 in, 2 out]
                    n2439 = property on="Start" class="Bool (strict)"("Visible"=FALSE, "DisabledEnum"=T7."Disabled and Grayed Out" ("Disabled")) -> ()  [unwired: 2 in, 2 out]
                  }
                  frame True {
                  }
                }
                n2440 = property on="Sampling rate" class="DigNum (strict)"("Visible"=FALSE, "DisabledEnum"=T7."Disabled" ("Disabled")) -> ()  [unwired: 2 in, 2 out]
              }
              frame "Lifetime (scan)" {
                w5738 = T7."Disabled" ("Disabled")
                w5737 = FALSE ("Visible")
                n2441 = call "lifetimeparameters.vi"("command"="get") -> ("Params out"=w5750:T22)  [unwired: 1 in]
                n2442 = local write "graphtab"(T8."image" ("graphtab")) -> ()
                n2443 = local write "Save tab"(enum32{"withsave", "withoutsave"}."withsave" ("Save tab")) -> ()
                n2444 = local write "Meastab"(enum32{"X-Y Image", "Linescan", "Timetrace"}."X-Y Image" ("Meastab")) -> ()
                n2445 = local write "Zscantab"(enum32{"withzscan", "withoutzscan", "lifetime"}."lifetime" ("Zscantab")) -> ()
                n2446 = Unbundle By Name(w5750) -> ("initialized"=w5749:bool)
                n2447 = property on="ttt" class="Enum (strict)"("Visible"=FALSE) -> ()  [unwired: 2 in, 2 out]
                n2448 = property on="refreshtime" class="DigNum (strict)"("Visible"=FALSE, "DisabledEnum"=T7."Disabled and Grayed Out" ("Disabled")) -> ()  [unwired: 2 in, 2 out]
                n2449 = property on="Pel" class="DigNum (strict)"("Visible"=w5737, "DisabledEnum"=w5738) -> ()  [unwired: 2 in, 2 out]
                n2450 = property on="bin" class="DigNum (strict)"("Visible"=w5737, "DisabledEnum"=w5738) -> ()  [unwired: 2 in, 2 out]
                n2451 = property on="save data" class="Bool (strict)"("Visible"=TRUE, "DisabledEnum"=T7."Enabled" ("Disabled"), "Value"=TRUE ("Visible")) -> ()  [unwired: 2 in, 2 out]
                n2452 = case shown="False" w5749 {
                  frame False {
                    n2453 = property on="Init" class="Bool (strict)"("Visible"=TRUE, "DisabledEnum"=T7."Enabled" ("Disabled")) -> ()  [unwired: 2 in, 2 out]
                    n2454 = property on="Start" class="Bool (strict)"("Visible"=FALSE, "DisabledEnum"=T7."Disabled and Grayed Out" ("Disabled")) -> ()  [unwired: 2 in, 2 out]
                  }
                  frame True {
                  }
                }
                n2455 = call "2pparameters.vi"("command"="get") -> ("params out"=w5755:T12)  [unwired: 1 in]
                n2456 = property on="continuous" class="Bool (strict)"("Visible"=TRUE, "DisabledEnum"=T7."Disabled and Grayed Out" ("Disabled")) -> ()  [unwired: 2 in, 2 out]
                n2457 = property on="finite samples" class="Bool (strict)"("Visible"=TRUE, "DisabledEnum"=T7."Enabled" ("Disabled")) -> ()  [unwired: 2 in, 2 out]
                n2458 = Bundle By Name(cluster=w5755, "type"="Lifetime (scan)") -> (w5753:T12)
                n2459 = call "2pparameters.vi"("Params in"=w5753, "command"="set") -> ()  [unwired: 1 out]
                n2460 = property on="finite samples" class="Bool (strict)"("Val(Sgnl)"=TRUE ("continuous for display")) -> ()  [unwired: 2 in, 2 out]
                n2461 = property on="continuous" class="Bool (strict)"("Value"=FALSE ("continuous for display")) -> ()  [unwired: 2 in, 2 out]
                n2462 = property on="srateAODOtt" class="DigNum (strict)"("Visible"=FALSE, "DisabledEnum"=T7."Disabled" ("Disabled")) -> ()  [unwired: 2 in, 2 out]
                n2463 = property on="# of frames" class="DigNum (strict)"("DisabledEnum"=T7."Enabled" ("Disabled"), "Caption.Text"="# of frames") -> ()  [unwired: 2 in, 2 out]
                n2464 = property on="img_CH1" class="IntGraph (strict)"("ZScale.Maximum"=12.5 ("Z Scale.Range:Maximum")) -> ()  [unwired: 2 in, 2 out]
                n2465 = property on="Current Average" class="DigNum (strict)"("Visible"=TRUE, "DisabledEnum"=T7."Enabled" ("Disabled")) -> ()  [unwired: 2 in, 2 out]
                n2466 = property on="Sampling rate" class="DigNum (strict)"("Visible"=TRUE, "DisabledEnum"=T7."Enabled" ("Disabled")) -> ()  [unwired: 2 in, 2 out]
                n2467 = property on="avpp" class="DigNum (strict)"("Visible"=TRUE, "DisabledEnum"=T7."Enabled" ("Disabled")) -> ()  [unwired: 2 in, 2 out]
              }
              frame "Lifetime (contour)" {
                w5779 = T7."Enabled" ("Disabled")
                w5778 = TRUE ("Visible")
                n2468 = call "2pparameters.vi"("command"="get") -> ("params out"=w5786:T12)  [unwired: 1 in]
                n2469 = property on="# of frames" class="DigNum (strict)"("DisabledEnum"=T7."Enabled" ("Disabled"), "Caption.Text"="# of samples") -> ()  [unwired: 2 in, 2 out]
                n2470 = property on="refreshtime" class="DigNum (strict)"("Visible"=TRUE, "DisabledEnum"=T7."Enabled" ("Disabled")) -> ()  [unwired: 2 in, 2 out]
                n2471 = Unbundle By Name(w5786) -> ("Angle draw"=w5788:dbl)
                n2472 = property on="avpp" class="DigNum (strict)"("Visible"=FALSE, "DisabledEnum"=T7."Disabled and Grayed Out" ("Disabled")) -> ()  [unwired: 2 in, 2 out]
                n2473 = property on="Current Average" class="DigNum (strict)"("Visible"=FALSE, "DisabledEnum"=T7."Disabled and Grayed Out" ("Disabled")) -> ()  [unwired: 2 in, 2 out]
                n2474 = local write "Angle drawing"(w5788) -> ()
                n2475 = local write "Save tab"(enum32{"withsave", "withoutsave"}."withsave" ("Save tab")) -> ()
                n2476 = local write "Zscantab"(enum32{"withzscan", "withoutzscan", "lifetime"}."lifetime" ("Zscantab")) -> ()
                n2477 = local write "graphtab"(T8."Lifetime" ("graphtab")) -> ()
                n2478 = local write "Meastab"(enum32{"X-Y Image", "Linescan", "Timetrace"}."Timetrace" ("Meastab")) -> ()
                n2479 = property on="ttt" class="Enum (strict)"("Visible"=TRUE) -> ()  [unwired: 2 in, 2 out]
                n2480 = call "lifetimeparameters.vi"("command"="get") -> ("Params out"=w5810:T22)  [unwired: 1 in]
                n2481 = property on="finite samples" class="Bool (strict)"("Val(Sgnl)"=TRUE ("continuous for display")) -> ()  [unwired: 2 in, 2 out]
                n2482 = local write "save\ndata"(TRUE ("save\ndata")) -> ()
                n2483 = Unbundle By Name(w5810) -> ("initialized"=w5811:bool)
                n2484 = property on="continuous" class="Bool (strict)"("Visible"=TRUE, "DisabledEnum"=T7."Enabled" ("Disabled")) -> ()  [unwired: 2 in, 2 out]
                n2485 = property on="finite samples" class="Bool (strict)"("Visible"=TRUE, "DisabledEnum"=T7."Enabled" ("Disabled")) -> ()  [unwired: 2 in, 2 out]
                n2486 = property on="Pel" class="DigNum (strict)"("Visible"=w5778, "DisabledEnum"=w5779) -> ()  [unwired: 2 in, 2 out]
                n2487 = property on="bin" class="DigNum (strict)"("Visible"=w5778, "DisabledEnum"=w5779) -> ()  [unwired: 2 in, 2 out]
                n2488 = property on="continuous" class="Bool (strict)"("Value"=FALSE ("continuous for display")) -> ()  [unwired: 2 in, 2 out]
                n2489 = case shown="False" w5811 {
                  frame False {
                    n2490 = property on="Init" class="Bool (strict)"("Visible"=TRUE, "DisabledEnum"=T7."Enabled" ("Disabled")) -> ()  [unwired: 2 in, 2 out]
                    n2491 = property on="Start" class="Bool (strict)"("Visible"=FALSE, "DisabledEnum"=T7."Disabled and Grayed Out" ("Disabled")) -> ()  [unwired: 2 in, 2 out]
                  }
                  frame True {
                  }
                }
                n2492 = property on="srateAODOtt" class="DigNum (strict)"("Visible"=TRUE, "DisabledEnum"=T7."Enabled" ("Disabled")) -> ()  [unwired: 2 in, 2 out]
                n2493 = call "2pparameters.vi"("command"="get") -> ("params out"=w5790:T12)  [unwired: 1 in]
                n2494 = Bundle By Name(cluster=w5790, "type"="Timetrace") -> (w5784:T12)
                n2495 = call "2pparameters.vi"("Params in"=w5784, "command"="set") -> ()  [unwired: 1 out]
                n2496 = property on="Sampling rate" class="DigNum (strict)"("Visible"=FALSE, "DisabledEnum"=T7."Disabled" ("Disabled")) -> ()  [unwired: 2 in, 2 out]
              }
            }
          }
          event "Laserpower  (%)": Value Change {
            n2497 = event-data() -> ("OldVal"=w5819:dbl, "NewVal"=w5820:dbl)  [unwired: 1 in, 4 out]
            n2498 = Not Equal?(x=w5819, y=w5820) -> (x != y?=w5821:bool)
            n2499 = case shown="True" w5821 {
              tunnel: w5820 -> [_ w5825]
              frame False {
              }
              frame True {
                n2500 = local read "wavelength(nm)"() -> (w5826:dbl)
                n2501 = call "configuration_2P_Linlin.vi"("command"="get") -> ("config out"=w5822:T14)  [unwired: 2 in, 1 out]
                n2502 = call "pockelscellcalibration.vi"("l"=w5826, "T"=w5825) -> ("Vout"=w5824:dbl)
                n2503 = Unbundle By Name(w5822) -> ("Vto2P"=w5829:i32, "AOlines"=w5828:tag[])
                n2504 = property on="lpow" class="DigNum (strict)"("Value"=w5825) -> ()  [unwired: 2 in, 2 out]
                n2505 = local write "Vpockels"(w5824) -> ()
                n2506 = Index Array(array=w5828, index=w5829) -> (element=w5827:tag)
                n2507 = call-poly <vilib>:"DAQmx Create Virtual Channel.vi"("physical channels"=w5827) -> ("task out"=w5831:refnum<k21>, "error out"=w5830:errorcluster)  [unwired: 13 in]
                n2508 = call-poly <vilib>:"DAQmx Write.vi"("task/channels in"=w5831, "data"=w5824, "error in"=w5830) -> ("task out"=w5832:refnum<k21>, "error out"=w5833:errorcluster)  [unwired: 10 in, 1 out]
                n2509 = call <vilib>:"DAQmx Start Task.vi"("task/channels in"=w5832, "error in"=w5833) -> ("task out"=w5834:refnum<k21>, "error out"=w5835:errorcluster)  [unwired: 12 in]
                n2510 = call <vilib>:"DAQmx Stop Task.vi"("task/channels in"=w5834, "error in"=w5835) -> ("task out"=w5836:refnum<k21>, "error out"=w5837:errorcluster)  [unwired: 12 in]
                n2511 = call <vilib>:"DAQmx Clear Task.vi"("task in"=w5836, "error in"=w5837) -> ()  [unwired: 13 in, 1 out]
              }
            }
          }
          event "lpow": Value Change {
            n2512 = event-data() -> ("OldVal"=w5838:dbl, "NewVal"=w5839:dbl)  [unwired: 1 in, 4 out]
            n2513 = Not Equal?(x=w5838, y=w5839) -> (x != y?=w5840:bool)
            n2514 = case shown="True" w5840 {
              tunnel: w5839 -> [_ w5845]
              frame False {
              }
